vi "lfs_read.vi"(8 "error in (no error)":errorcluster, 9 "initialize":bool, 11 "lfs ref in":refnum<class "IR sensor.lvclass">[](array[class])) -> (0 "error out":errorcluster, 1 "dbl Scaled Value left":dbl, 2 "dbl Scaled Value right":dbl, 3 "lfs ref":refnum<class "IR sensor.lvclass">[](array[class]))   [LabVIEW 2019]
uses:
  FPGA_subVIs/low level/IR sensor/IR sensor.lvclass
  <vilib>/ptbypt/NI_PtbyPt.lvlib
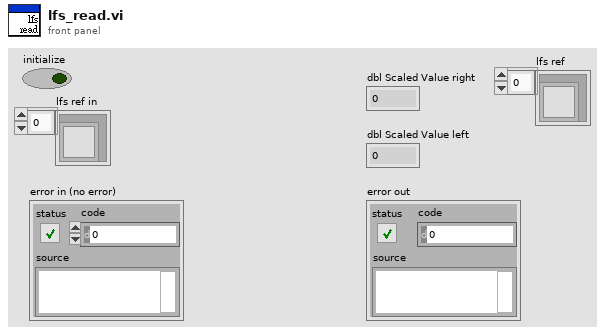
[diagram p1: front panel]
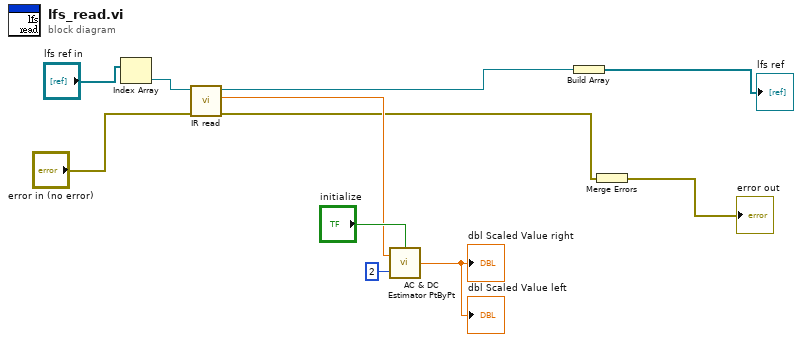
[diagram p0: block diagram]
diagram:
  n1 = Index Array(array="lfs ref in") -> (element=w8:refnum<class "IR sensor.lvclass">)  [unwired: 1 in]
  n2 = call-dynamic "IR read.vi"("error in (no error)"="error in (no error)", "IR sensor in"=w8) -> ("error out"=w4:errorcluster, "IR"=w6:dbl, "IR sensor out"=w5:refnum<class "IR sensor.lvclass">)  [unwired: 7 in]
  n3 = call <vilib>:"AC & DC Estimator PtByPt.vi"("signal"=w6, "sample length"=2, "initialize"="initialize") -> ("DC estimate (V)"=→"dbl Scaled Value right" →"dbl Scaled Value left":dbl)  [unwired: 2 out]
  n4 = Build Array(w5) -> (→"lfs ref":refnum<class "IR sensor.lvclass">[])
  n5 = Merge Errors(w4) -> (→"error out":errorcluster)
